vi "AddLimit.vi"(7 "ComparisonType":T1, 8 "error in":errorcluster, 9 "HigherBond":dbl, 10 "LowerBound":dbl, 11 "RealMeasure in":refnum<class "RealMeasure.lvclass">) -> (0 "error out":errorcluster, 2 "RealMeasureLimit":refnum<class "RealMeasureLimit.lvclass">, 3 "RealMeasure out":refnum<class "RealMeasure.lvclass">)   [LabVIEW 2021, in "ProligentXMLGenerator.lvlib" / "RealMeasure.lvclass"]
doc: "Add a MeasureLimit element.\n\nThe limit expression associated with the measure."
uses:
  RealMeasure.lvclass
  RealMeasure.lvclass/RealMeasure.ctl
  MeasureLimit/MeasureLimit.lvclass
  RealMeasureLimit/RealMeasureLimit.lvclass
  RangeMeasureLimit/ComparisonType.ctl
  RangeMeasureLimit/RangeMeasureLimit.lvclass
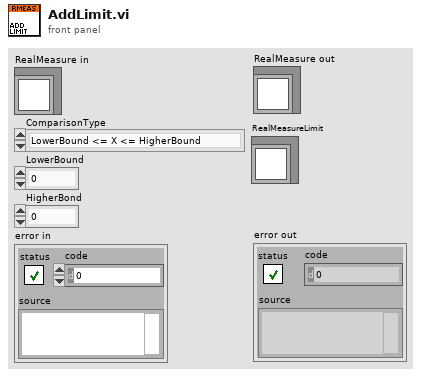
[diagram p1: front panel]
types:
  T1 = typedef "ProligentXMLGenerator.lvlib/RangeMeasureLimit.lvclass/ComparisonType.ctl" = enum16{"LowerBound <= X <= HigherBound", "LowerBound < X <= HigherBound", "LowerBound <= X < HigherBound", "LowerBound < X < HigherBound", "LowerBound <= X", "LowerBound < X", "X <= HigherBound", "X < HigherBound", "X == HigherBound", "X != HigherBound", "X <= LowerBound OR HigherBound <= X", "X < LowerBound OR HigherBound <= X", "X <= LowerBound OR HigherBound < X", "X < LowerBound OR HigherBound < X"}
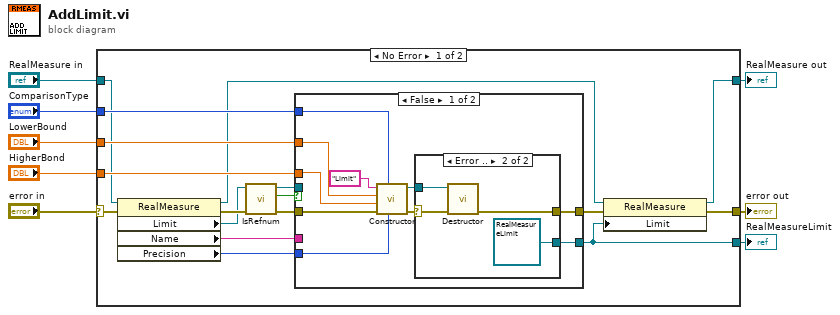
[diagram p0: block diagram]
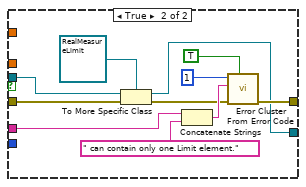
[diagram p3: hidden frame]
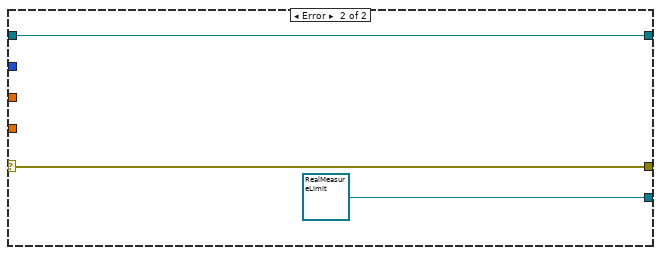
[diagram p4: hidden frame]
diagram:
  n1 = case shown="No Error" "error in" {
    selector: "error in" -> [w24 w54]
    tunnel: [w13 refnum<class "RealMeasureLimit.lvclass"> refnum ("ProligentResultProcessor:RealMeasureLimit")] -> w4
    tunnel: [w15 w54] -> w7
    tunnel: "RealMeasure in" -> [w12 w55]
    tunnel: [w14 w55] -> w5
    tunnel: "ComparisonType" -> [w19 _]
    tunnel: "LowerBound" -> [w18 _]
    tunnel: "HigherBond" -> [w17 _]
    frame No Error {
      n2 = property class="RealMeasure"(reference=w12, error in=w24) -> (reference out=w11:refnum<class "RealMeasure.lvclass">, error out=w23:errorcluster, "Limit"=w10:refnum<class "MeasureLimit.lvclass">, "Name"=w22:string, "Precision"=w16:u8)
      n3 = call "IsRefnum.vi"("error in"=w23, "MeasureLimit in"=w10) -> ("error out"=w21:errorcluster, "IsRefnum"=w20:bool, "MeasureLimit out"=w9:refnum<class "MeasureLimit.lvclass">)  [unwired: 7 in]
      n4 = case shown="False" w20 {
        tunnel: w21 -> [w28 w45]
        tunnel: [w35 w48] -> w25
        tunnel: [w34 w43] -> w13
        tunnel: w22 -> [_ w47]
        tunnel: w19 -> [w33 _]
        tunnel: w18 -> [w32 _]
        tunnel: w17 -> [w30 _]
        tunnel: w16 -> [w29 _]
        tunnel: w9 -> [_ w46]
        frame False {
          n5 = call "Constructor.vi"("Precision"=w29, "ComparisonType"=w33, "error in"=w28, "HigherBond"=w30, "LowerBound"=w32, "Name"="Limit") -> ("error out"=w27:errorcluster, "RealMeasureLimit"=w26:refnum<class "RealMeasureLimit.lvclass">)  [unwired: 4 in]
          n6 = case shown="Error .." w27 {
            selector: w27 -> [w36 w41]
            tunnel: w26 -> [w37 w39]
            tunnel: [w36 w40] -> w35
            tunnel: [w37 refnum<class "RealMeasureLimit.lvclass"> refnum ("ProligentResultProcessor:RealMeasureLimit")] -> w34
            frame No Error {
            }
            frame Error {
              n7 = call "Destructor.vi"("error in"=w41, "RealMeasureLimit"=w39) -> ("error out"=w40:errorcluster)  [unwired: 9 in]
            }
          }
        }
        frame True {
          n8 = To More Specific Class(target class=refnum<class "RealMeasureLimit.lvclass"> refnum ("ProligentResultProcessor:RealMeasureLimit"), reference=w46, error in=w45) -> (specific class reference=w43:refnum<class "RealMeasureLimit.lvclass">, error out=w44:errorcluster)
          n9 = Concatenate Strings(w47, " can contain only one Limit element." ("string")) -> (w52:string)
          n10 = call <vilib>:"Error Cluster From Error Code.vi"("show call chain? (False)"=TRUE, "error in (no error)"=w44, "error message (\"\")"=w52, "error code (0)"=1) -> ("error out"=w48:errorcluster)  [unwired: 5 in]
        }
      }
      n11 = property class="RealMeasure"(reference=w11, error in=w25, "Limit"=w13) -> (reference out=w14:refnum<class "RealMeasure.lvclass">, error out=w15:errorcluster)
    }
    frame Error {
    }
  }
  "error out" <- w7
  "RealMeasure out" <- w5
  "RealMeasureLimit" <- w4
